vi "电缸参数.vi"(8 "写入数据":u32, 9 "写入地址":u32=22, 10 "枚举":enum16{"读取", "写入"}(ring)) -> (3 "拉压测试状态":dbl format="%#_4g")   [LabVIEW 2020]
uses:
  S7/S7Ref.vi
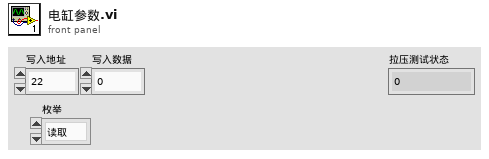
[diagram p1: front panel]
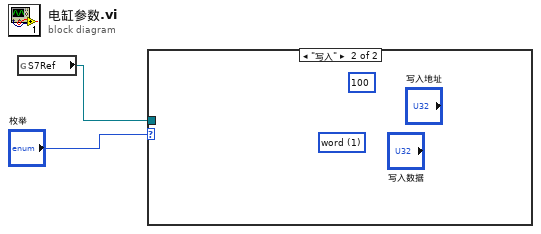
[diagram p0: block diagram]
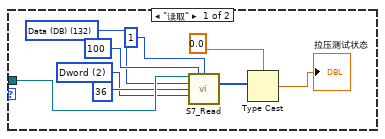
[diagram p2: hidden frame]
diagram:
  n1 = global read "S7Ref.vi" "S7Ref"() -> (w1:refnum<k5>)
  n2 = case shown="\"写入\"" "枚举" {
    tunnel: w1 -> [w8 _]
    frame "读取" {
      w5 = u8 132 items=["I/O (P)"=128, "Input (I)"=129, "Output (Q)"=130, "Bit Memory (M)"=131, "Data (DB)"=132, "Instance Data (DI)"=133, "Local Data (L)"=134, "Predecessor Local Data (VL)"=135] ("寄存器类型")
      w3 = u16 2 items=["byte", "word", "Dword"] ("数据类型")
      n3 = call "S7_Read.vi"("TCP"=w8, "DB #"=u16 100, "读取长度"=u16 1, "寄存器类型"=w5, "起始地址"=u32 36, "数据类型"=w3) -> ("数据"=w11:u32[])  [unwired: 6 in, 3 out]
      n4 = Type Cast(type=0.0, x=w11) -> (*(type *) &x=→"拉压测试状态":dbl)
    }
    frame "写入" {
      (unwired) u16 1 items=["byte", "word", "Dword"] ("数据类型")
      (unwired) u16 100 ("DB #")
    }
  }
